vi "Read Config File (SubVI).vi"(0 "configuration file path":path=path "C:/Projet_CETAL_DESY_CSCI/POSTES LOCAUX/PROJECT_GAIA_HP/Development/Config/User.ini" caption="chemin du fichier de configuration", 5 "entrée d'erreur (pas d'erreur)":errorcluster) -> (14 "file path":path, 15 "User file contents Energie UV":dbl[](array[numeric]), 16 "User file contents Energie IR":dbl[](array[numeric]), 17 "User file contents Puissance depolar":dbl[](array[numeric]), 18 "error?":bool caption="erreur ?", 19 "sortie d'erreur":errorcluster)   [LabVIEW 2017]
uses:
  <vilib>/Utility/config.llb/Read Key (String).vi
  <vilib>/Utility/config.llb/NI_LVConfig.lvlib
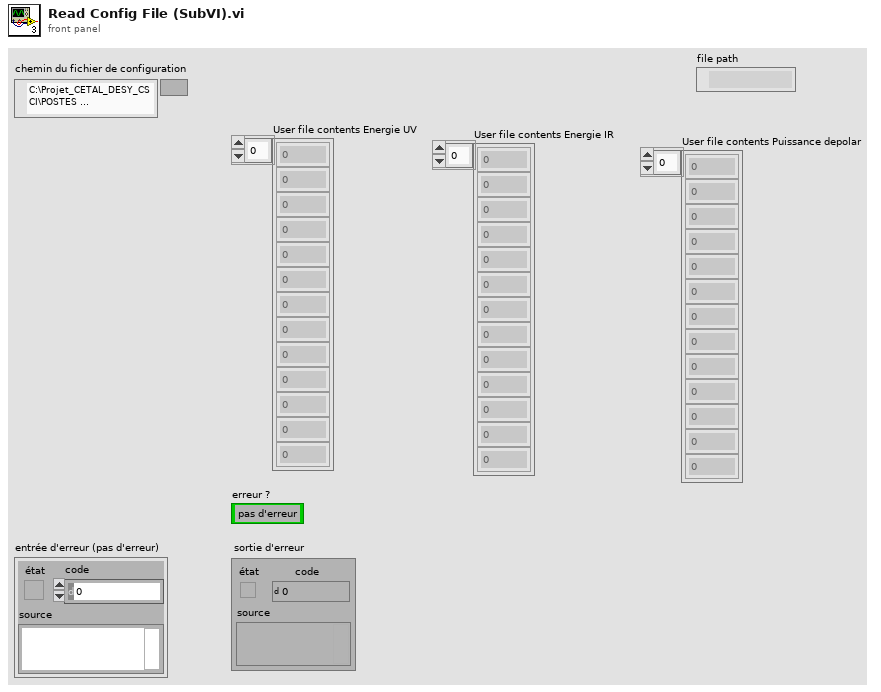
[diagram p1: front panel]
types:
  T1 = typedef "NI_LVConfig.lvlib/Config Data RefNum.ctl" = refnum<k1>
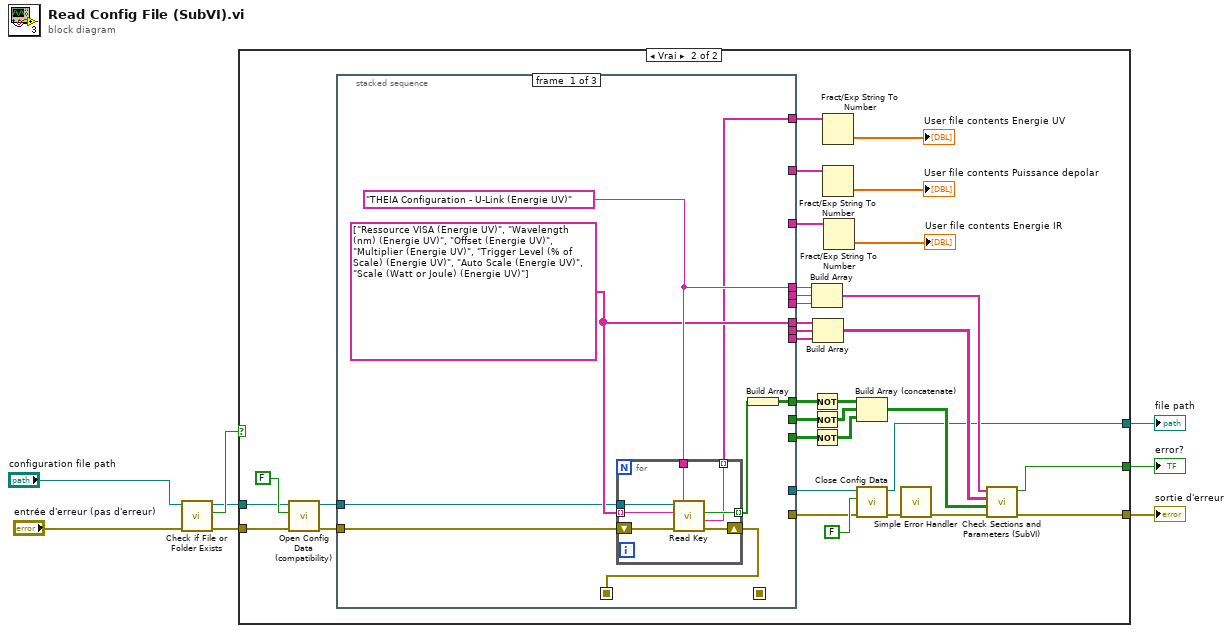
[diagram p0: block diagram]
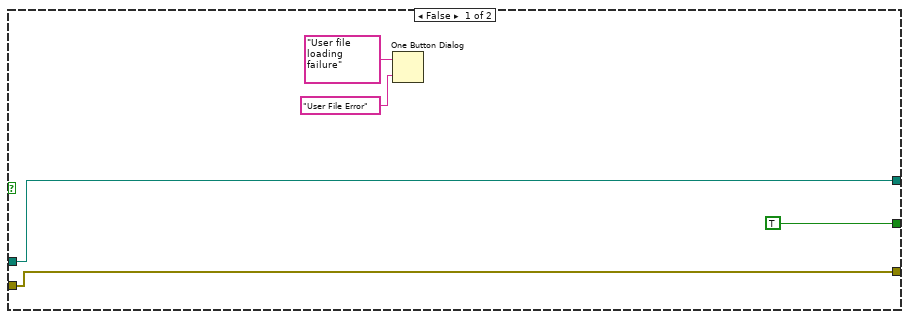
[diagram p2: hidden frame]
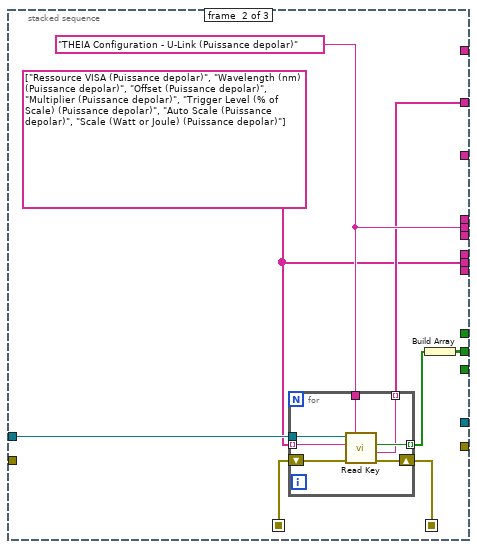
[diagram p3: hidden frame]
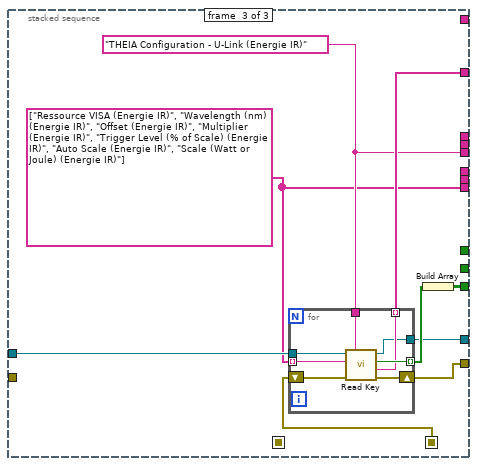
[diagram p4: hidden frame]
diagram:
  n1 = call <vilib>:"Check if File or Folder Exists.vi"("error in (no error)"="entrée d'erreur (pas d'erreur)", "path"="configuration file path") -> ("error out"=w5:errorcluster, "file or folder exists?"=w8:bool, "dup path"=w6:path)  [unwired: 7 in]
  n2 = case shown="Vrai" w8 {
    tunnel: w6 -> [w9 w43]
    tunnel: w5 -> [w11 w40]
    tunnel: [w11 w31] -> w3
    tunnel: [TRUE ("Erreur ?") w30] -> w4
    tunnel: [w9 w14] -> w1
    frame False {
      n3 = One Button Dialog(message="User file loading failure" ("Line1_message"), button name ("OK")="User File Error" ("Title")) -> ()  [unwired: 1 out]
    }
    frame True {
      n4 = call <vilib>:"Open Config Data (compatibility).vi"("error in (no error)"=w40, "create file if necessary (T)"=FALSE ("create file if necessary? (T)"), "configuration file path"=w43) -> ("error out"=w46:errorcluster, "refnum"=w41:T1)  [unwired: 6 in, 1 out]
      n5 = stacked-sequence {
        seq-local: [w54 _ _] -> [_ w69 _]
        seq-local: [_ w64 _] -> [_ _ w80]
        tunnel: w46 -> [w55 _ _]
        tunnel: w41 -> [w50 w70 w86]
        tunnel: [_ _ w85] -> w42
        tunnel: [w53 _ _] -> w39
        tunnel: [_ w66 _] -> w38
        tunnel: [w51 _ _] -> w37
        tunnel: [_ w63 _] -> w36
        tunnel: [w48 _ _] -> w35
        tunnel: [_ w67 _] -> w34
        tunnel: [_ _ w79] -> w25
        tunnel: [w49 _ _] -> w23
        tunnel: [_ w65 _] -> w21
        tunnel: [_ _ w83] -> w19
        tunnel: [_ _ w82] -> w18
        tunnel: [_ _ w78] -> w17
        tunnel: [_ _ w81] -> w15
        frame #0 {
          w51 = string[] ["Ressource VISA (Energie UV)", "Wavelength (nm) (Energie UV)", "Offset (Energie UV)", "Multiplier (Energie UV)", "Trigger Level (% of Scale) (Energie UV)", "Auto Scale (Energie UV)", "Scale (Watt or Joule) (Energie UV)"]
          w53 = "THEIA Configuration - U-Link (Energie UV)" ("section")
          n6 = for {
            shift-right: [w61] -> w54
            shift-left: w55 -> [w62]
            tunnel: w53 -> [w60]
            tunnel: w51 -> [w59] mode=indexing
            tunnel: w50 -> [w58]
            tunnel: [w57] -> w52 mode=indexing
            tunnel: [w56] -> w49 mode=indexing
            n7 = call-poly <vilib>:"Read Key.vi"("section"=w60, "error in (no error)"=w62, "key"=w59, "refnum"=w58) -> ("error out"=w61:errorcluster, "value"=w56:string, "found?"=w57:bool)  [unwired: 2 in, 3 out]
          }
          n8 = Build Array(w52) -> (w48:bool[][])
        }
        frame #1 {
          w63 = string[] ["Ressource VISA (Puissance depolar)", "Wavelength (nm) (Puissance depolar)", "Offset (Puissance depolar)", "Multiplier (Puissance depolar)", "Trigger Level (% of Scale) (Puissance depolar)", "Auto Scale (Puissance depolar)", "Scale (Watt or Joule) (Puissance depolar)"]
          w66 = "THEIA Configuration - U-Link (Puissance depolar)" ("section")
          n9 = for {
            shift-right: [w76] -> w64
            shift-left: w69 -> [w77]
            tunnel: w66 -> [w75]
            tunnel: w63 -> [w74] mode=indexing
            tunnel: w70 -> [w73]
            tunnel: [w72] -> w68 mode=indexing
            tunnel: [w71] -> w65 mode=indexing
            n10 = call-poly <vilib>:"Read Key.vi"("section"=w75, "error in (no error)"=w77, "key"=w74, "refnum"=w73) -> ("error out"=w76:errorcluster, "value"=w71:string, "found?"=w72:bool)  [unwired: 2 in, 3 out]
          }
          n11 = Build Array(w68) -> (w67:bool[][])
        }
        frame #2 {
          w78 = string[] ["Ressource VISA (Energie IR)", "Wavelength (nm) (Energie IR)", "Offset (Energie IR)", "Multiplier (Energie IR)", "Trigger Level (% of Scale) (Energie IR)", "Auto Scale (Energie IR)", "Scale (Watt or Joule) (Energie IR)"]
          w82 = "THEIA Configuration - U-Link (Energie IR)" ("section")
          n12 = for {
            shift-right: [w93] -> w85
            shift-left: w80 -> [w94]
            tunnel: w82 -> [w92]
            tunnel: w78 -> [w91] mode=indexing
            tunnel: w86 -> [w90]
            tunnel: [w89] -> w84 mode=indexing
            tunnel: [w88] -> w83 mode=indexing
            tunnel: [w87] -> w79
            n13 = call-poly <vilib>:"Read Key.vi"("section"=w92, "error in (no error)"=w94, "key"=w91, "refnum"=w90) -> ("error out"=w93:errorcluster, "value"=w88:string, "found?"=w89:bool, "refnum out"=w87:T1)  [unwired: 2 in, 2 out]
          }
          n14 = Build Array(w84) -> (w81:bool[][])
        }
      }
      n15 = Build Array(w39, w38, w18) -> (w29:string[])
      n16 = Not(x=w35) -> (.not. x?=w33:bool[][])
      n17 = Not(x=w34) -> (.not. x?=w32:bool[][])
      n18 = Not(x=w15) -> (.not. x?=w16:bool[][])
      n19 = Build Array(w37, w36, w17) -> (w28:string[][])
      n20 = Fract/Exp String To Number(string=w23) -> (number=→"User file contents Energie UV":dbl[])  [unwired: 3 in, 1 out]
      n21 = Fract/Exp String To Number(string=w21) -> (number=→"User file contents Puissance depolar":dbl[])  [unwired: 3 in, 1 out]
      n22 = Fract/Exp String To Number(string=w19) -> (number=→"User file contents Energie IR":dbl[])  [unwired: 3 in, 1 out]
      n23 = Build Array (concatenate)(w33, w32, w16) -> (w27:bool[][])
      n24 = call <vilib>:"Close Config Data.vi"("error in (no error)"=w42, "write file if changed (T)"=FALSE ("write configuration file? (T)"), "refnum"=w25) -> ("error out"=w45:errorcluster, "file path"=w14:path)  [unwired: 7 out]
      n25 = call <vilib>:"Simple Error Handler.vi"("error in (no error)"=w45) -> ("error out"=w26:errorcluster)  [unwired: 1 in, 7 out]
      n26 = call "Check Sections and Parameters (SubVI).vi"("entrée d'erreur (pas d'erreur)"=w26, "found? array"=w27, "Parameter array"=w28, "Section array"=w29) -> ("sortie d'erreur"=w31:errorcluster, "Erreur ?"=w30:bool)  [unwired: 6 in]
    }
  }
  "error?" <- w4
  "sortie d'erreur" <- w3
  "file path" <- w1
